vi "PH_gentec_Powermeter.evt call Set Statistics Config.vi"(0 "i ref in":refnum<vi>, 2 "Instance":string, 3 "Number Of Pulses":T1={"Sample Rate"=10, "Sample Rate Unit"=100, "Sample Period"=20, "Sample Period Unit"=0, "Total Duration"=0, "Total Duration Unit"=0, "Time Stamp"=0} {"Time Stamp" items=["Off", "On"]; "Total Duration Unit" items=["Period", "Seconds", "Minutes", "Hours", "Days", "Weeks", "Continuous", "# of Points"]; "Total Duration" max=300 step=1; "Sample Period Unit" items=["Seconds", "Minutes", "Hours", "Days", "Weeks", "Pulses"]; "Sample Rate Unit" items=["per Second", "per Minute", "per Hour", "per Day", "% pulses"]; "Sample Rate" max=300 step=1}, 5 "error in (no error)":errorcluster) -> (14 "i ref out":refnum<vi>, 19 "error out":errorcluster)   [LabVIEW 2014, in "PH_gentec_Powermeter.lvlib"]
doc: "This VI sets the number of pulses by a simple call."
uses:
  PH_gentec_Powermeter.lvlib
  non_GPL/instr.lib/gentec-SOLO-PE/Driver/Type Defs/gentec-SOLO-PE.Data Sampling Settings.ctl
  CSCore/CSSystem/CoreLib/CoreLib.int 2 byte array.vi
  CSCore/CSSystem/CoreLib/CoreLib.lvlib
  CSCore/BaseProcess/BaseProcess.lvlib
  non_GPL/instr.lib/gentec-SOLO-PE/gentec-SOLO-PE - Driver.lvlib
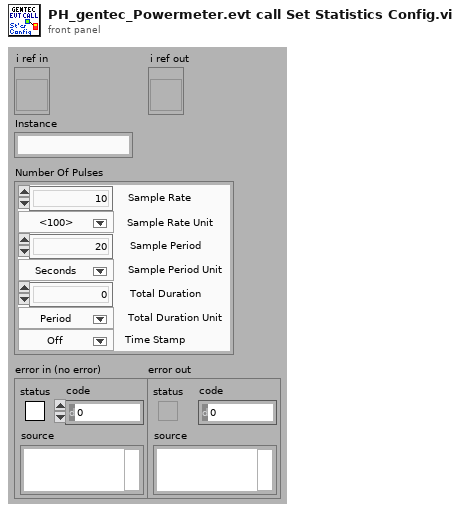
[diagram p1: front panel]
types:
  T1 = typedef "gentec-SOLO-PE - Driver.lvlib/gentec-SOLO-PE.Data Sampling Settings.ctl" = cluster{"Sample Rate":u32, "Sample Rate Unit":u32, "Sample Period":u32, "Sample Period Unit":u32, "Total Duration":u32, "Total Duration Unit":u32, "Time Stamp":u32}
  T2 = typedef "CoreDefs.rawDataType.ctl" = i8[]
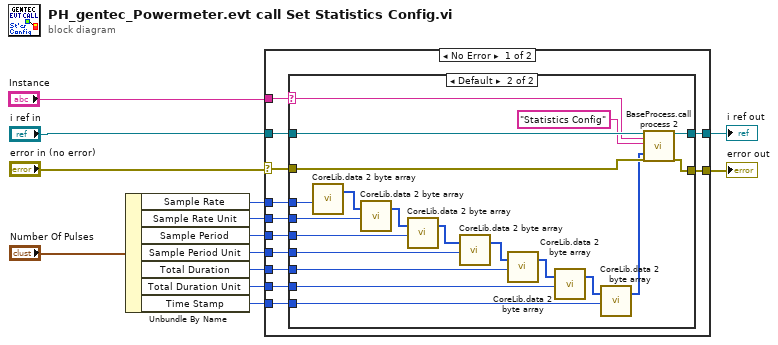
[diagram p0: block diagram]
diagram:
  n1 = Unbundle By Name("Number Of Pulses") -> ("Sample Rate"=w7:u32, "Sample Rate Unit"=w6:u32, "Sample Period"=w5:u32, "Sample Period Unit"=w4:u32, "Total Duration"=w3:u32, "Total Duration Unit"=w2:u32, "Time Stamp"=w1:u32)
  n2 = case shown="No Error" "error in (no error)" {
    selector: "error in (no error)" -> [w20 w48]
    tunnel: [w25 w49] -> w9
    tunnel: [w24 w48] -> w8
    tunnel: "i ref in" -> [w23 w49]
    tunnel: "Instance" -> [w21 _]
    tunnel: w7 -> [w22 _]
    tunnel: w6 -> [w19 _]
    tunnel: w5 -> [w18 _]
    tunnel: w4 -> [w17 _]
    tunnel: w3 -> [w16 _]
    tunnel: w2 -> [w15 _]
    tunnel: w1 -> [w14 _]
    frame No Error {
      n3 = case shown="Default" w21 {
        selector: w21 -> [_ w41]
        tunnel: [w27 w47] -> w25
        tunnel: [w26 w46] -> w24
        tunnel: w23 -> [w27 w45]
        tunnel: w20 -> [w26 w44]
        tunnel: w22 -> [_ w42]
        tunnel: w19 -> [_ w40]
        tunnel: w18 -> [_ w39]
        tunnel: w17 -> [_ w33]
        tunnel: w16 -> [_ w32]
        tunnel: w15 -> [_ w31]
        tunnel: w14 -> [_ w30]
        frame "N/A" {
        }
        frame Default {
          n4 = call-poly "CoreLib.data 2 byte array.vi"("i32"=w42) -> ("byteArray out"=w38:T2)  [unwired: 18 in]
          n5 = call-poly "CoreLib.data 2 byte array.vi"("byteArray"=w38, "i32"=w40) -> ("byteArray out"=w37:T2)  [unwired: 17 in]
          n6 = call-poly "CoreLib.data 2 byte array.vi"("byteArray"=w37, "i32"=w39) -> ("byteArray out"=w34:T2)  [unwired: 17 in]
          n7 = call-poly "CoreLib.data 2 byte array.vi"("byteArray"=w34, "i32"=w33) -> ("byteArray out"=w36:T2)  [unwired: 17 in]
          n8 = call-poly "CoreLib.data 2 byte array.vi"("byteArray"=w36, "i32"=w32) -> ("byteArray out"=w35:T2)  [unwired: 17 in]
          n9 = call-poly "CoreLib.data 2 byte array.vi"("byteArray"=w35, "i32"=w31) -> ("byteArray out"=w29:T2)  [unwired: 17 in]
          n10 = call-poly "CoreLib.data 2 byte array.vi"("byteArray"=w29, "i32"=w30) -> ("byteArray out"=w28:T2)  [unwired: 17 in]
          n11 = call "BaseProcess.call process 2.vi"("i ref in"=w45, "Object"=w41, "Selector"="Statistics Config", "Data"=w28, "error in (no error)"=w44) -> ("i ref out"=w47:refnum<vi>, "error out"=w46:errorcluster)  [unwired: 13 in]
        }
      }
    }
    frame Error {
    }
  }
  "error out" <- w8
  "i ref out" <- w9
